vi "Query FTT Data.vi"(8 "error in (no error)":errorcluster, 11 "Main":T1={"Tite"="", "Base path"=path "", "Table"=[], "Stations"=[], "Shield Array"=[], "UPHs"=[], "VISA"={"VISA"="", "baud rate"=9600, "data bits"=8, "parity"=enum."None", "stop bits"=10, "flow control"=0}, "Path"={"roof"=path "", "Config"=path "", "Png"=path ""}, "Ctr"={"DB Dispaly"=refnum, "Error Table"=refnum, "Display"=refnum, "Login"=refnum, "Exit"=refnum, "FTT_Submit"=refnum}, "Login"={"User"="", "Grade"=""}, "information"={"cause"="", "Type"=enum."Inform", "code"=0, "Suroce"="", "Status"=FALSE}, "Local DB"={"Connstr"="", "Database"={"Constr"={"Driver"="", "Server"="", "User"="", "Pwd"="", "Database"=""}, "conn ref"=refnum, "State"=FALSE}}, "Remote DB"={"Connstr"="", "Database"={"Constr"={"Driver"="", "Server"="", "User"="", "Pwd"="", "Database"=""}, "conn ref"=refnum, "State"=FALSE}}, "FTT TV"="", "ExchangeTime"=0, "NVH"="", "EOL Path"=path ""} {"VISA"."flow control" items=["None", "XON/XOFF", "RTS/CTS", "XON/XOFF & RTS/CTS", "DTR/DSR", "XON/XOFF & DTR/DSR"]; "VISA"."stop bits" items=["1.0"=10, "1.5"=15, "2.0"=20]}) -> (0 "error out":errorcluster)   [LabVIEW 2014]
uses:
  Type'def/DB Query.ctl
  <vilib>/Utility/file.llb/Write Delimited Spreadsheet (string).vi
  Type'def/UPH Config.ctl
  VISA/Ctr/VISA Ctr.ctl
  Type'def/Main Ctr Ref.ctl
  Type'def/User Login.ctl
  Database/Ctr/Constr.ctl
  <vilib>/addons/database/Connection.llb/Conn ObjectReference.ctl
  <vilib>/addons/database/NI_Database_API.lvlib
  Database/Ctr/Conneect State.ctl
  Type'def/MainCtr.ctl
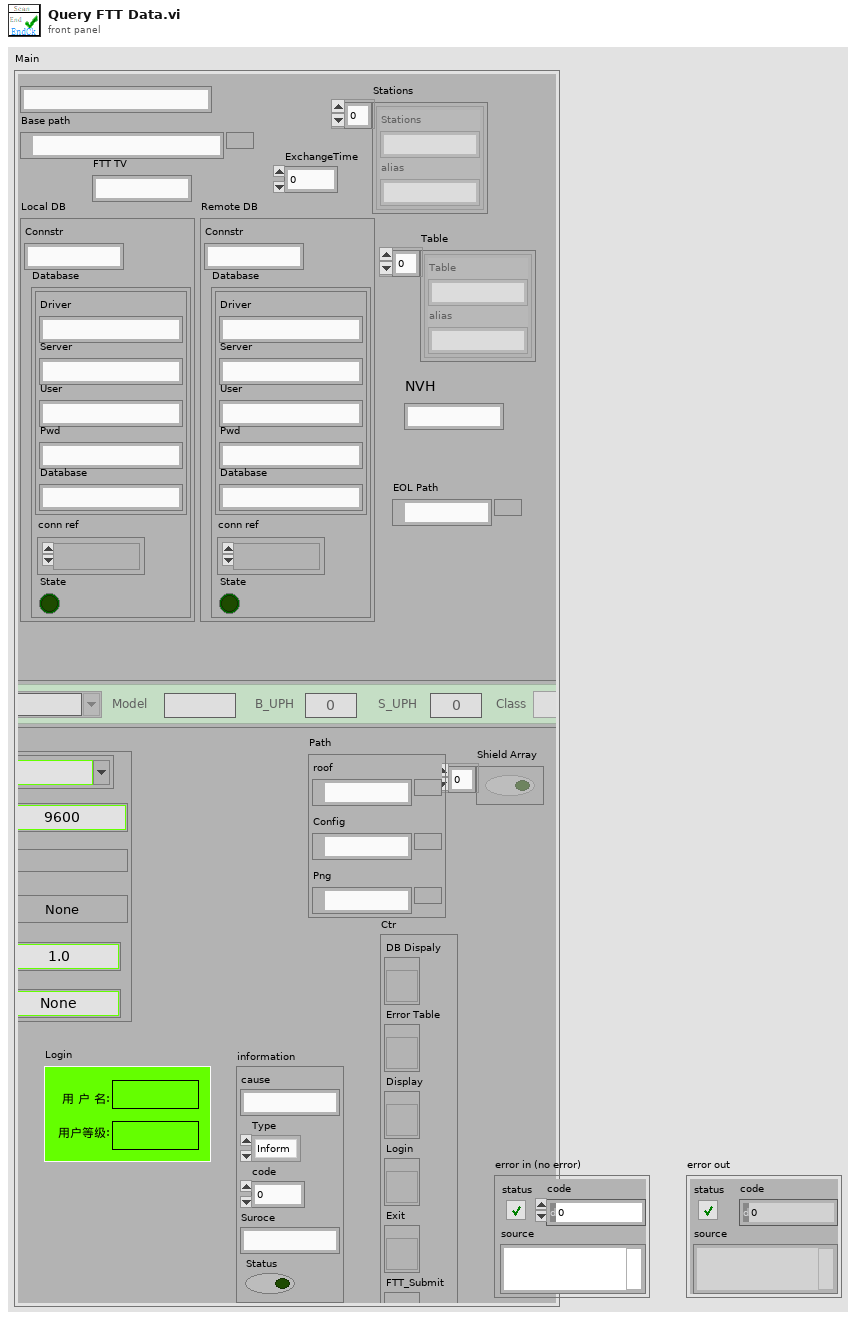
[diagram p1: front panel]
types:
  T1 = typedef "MainCtr.ctl" = cluster{"Tite":string, "Base path":path, "Table":cluster{"Table":string, "alias":string}[], "Stations":cluster{"Stations":string, "alias":string}[], "Shield Array":bool[], "UPHs":T2[], "VISA":T3, "Path":cluster{"roof":path, "Config":path, "Png":path}, "Ctr":T4, "Login":T5, "information":cluster{"cause":string, "Type":enum16{"Inform", "Warning", "Alarm"}, "code":i32, "Suroce":string, "Status":bool}, "Local DB":cluster{"Connstr":string, "Database":T6}, "Remote DB":cluster{"Connstr":string, "Database":T6}, "FTT TV":string, "ExchangeTime":i32, "NVH":string, "EOL Path":path}
  T2 = typedef "UPH Config.ctl" = cluster{"Line_No":string, "Model":string, "B_UPH ":i16, "S_UPH  ":i16, "Class":enum16{"Big", "Small"}}
  T3 = typedef "VISA Ctr.ctl" = cluster{"VISA":refnum<visa-resource-name>, "baud rate":u32, "data bits":u16, "parity":enum16{"None", "Odd", "Even", "Mark", "Space"}, "stop bits":u16, "flow control":u16}
  T4 = typedef "Main Ctr Ref.ctl" = cluster{"DB Dispaly":refnum<vi>, "Error Table":refnum<vi>, "Display":refnum<vi>, "Login":refnum<vi>, "Exit":refnum<vi>, "FTT_Submit":refnum<vi>}
  T5 = typedef "User Login.ctl" = cluster{"User":string, "Grade":string}
  T6 = typedef "Conneect State.ctl" = cluster{"Constr":T7, "conn ref":T8, "State":bool}
  T7 = typedef "Constr.ctl" = cluster{"Driver":string, "Server":string, "User":string, "Pwd":string, "Database":string}
  T8 = typedef "NI_Database_API.lvlib/Conn ObjectReference.ctl" = refnum<k1>
  T9 = cluster{"cause":string, "Type":enum16{"Inform", "Warning", "Alarm"}, "code":i32, "Suroce":string, "Status":bool}
  T10 = typedef "DB Query.ctl" = cluster{"Export":bool, "Query":bool, "Station.No":string, "EndTime":timestamp, "StartTime":timestamp, "FTT":cluster{"FTT":string, "OutLine":string, "FTT Rata":string}, "TableName":string, "List":string[][], "Station":bool, "QTime":enum32{"Online", "Outline"}}
  T11 = cluster{"Main ":T1, "DB Dispaly":T10, "information":cluster{"cause":string, "Type":enum16{"Inform", "Warning", "Alarm"}, "code":i32, "Suroce":string, "Status":bool}, "CmdStr":string, "OnlineStr":string}
  T12 = cluster{"FTT":string, "OutLine":string, "FTT Rata":string}
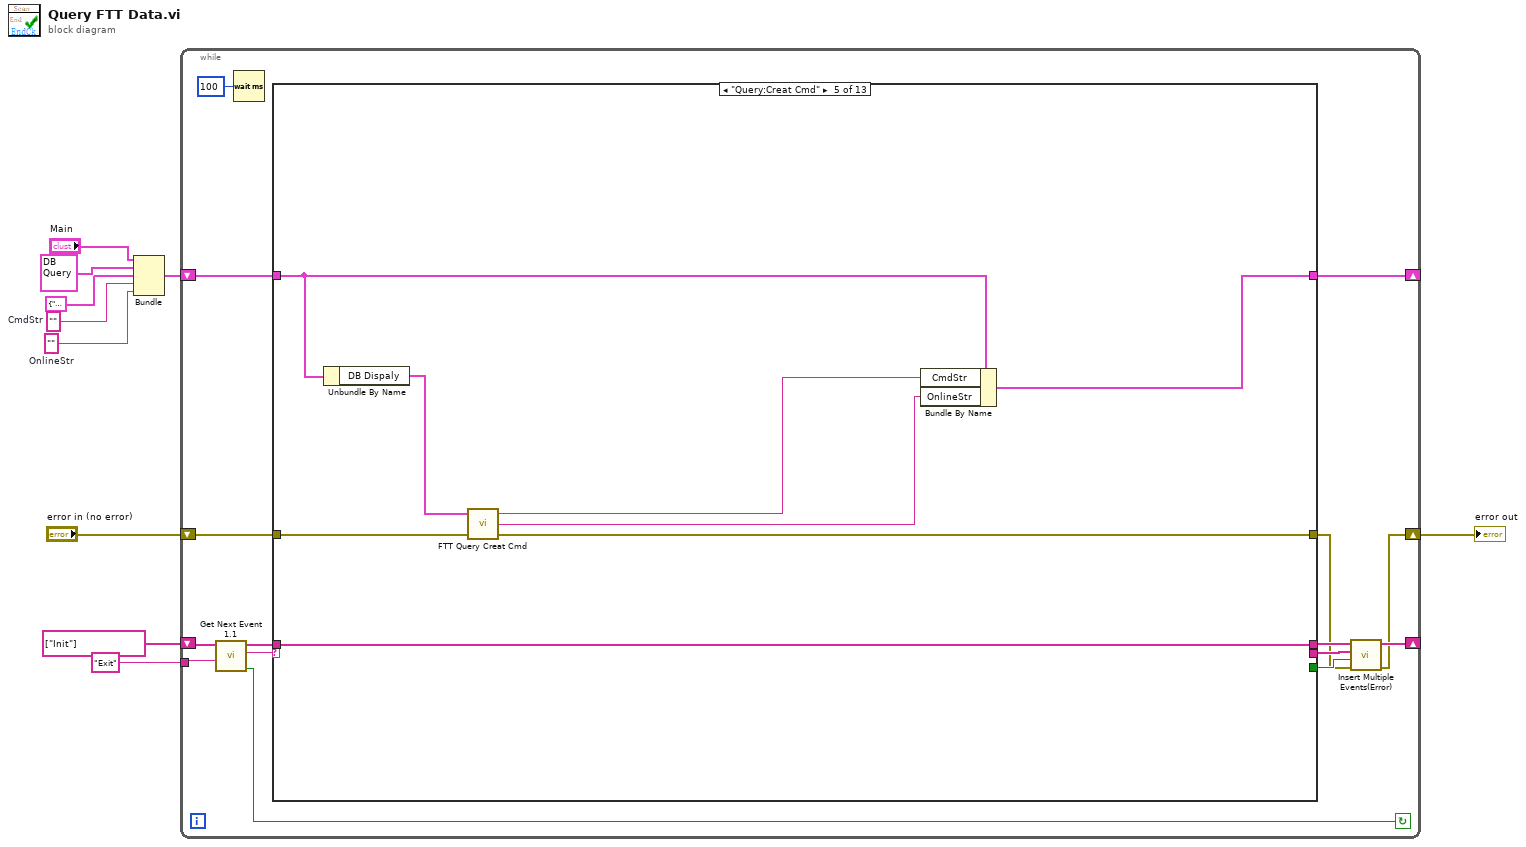
[diagram p0: block diagram]
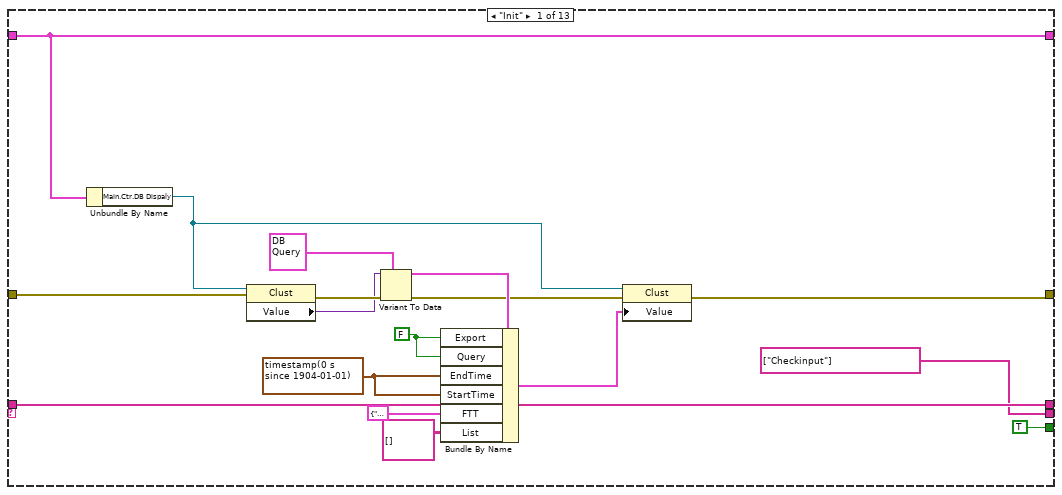
[diagram p2: hidden frame]
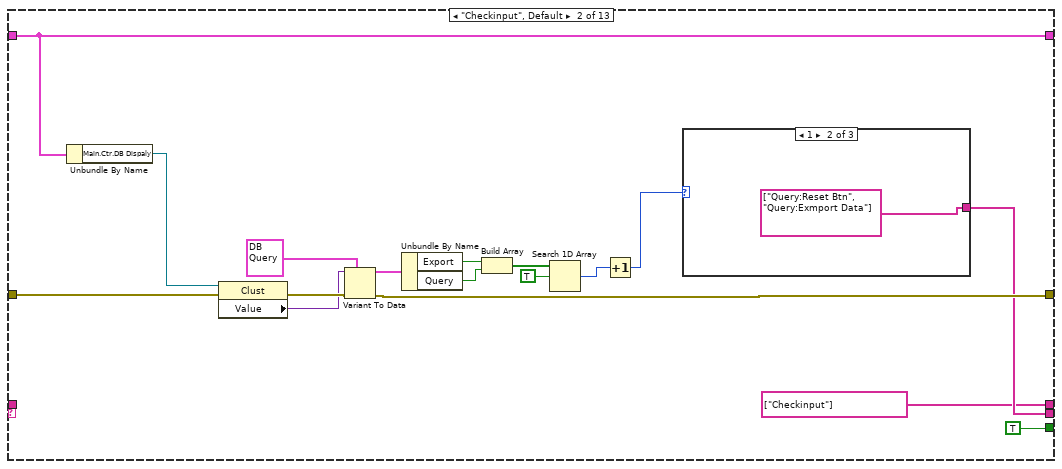
[diagram p3: hidden frame]
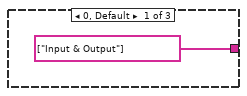
[diagram p4: hidden frame]
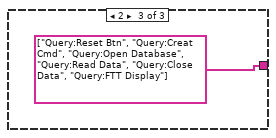
[diagram p5: hidden frame]
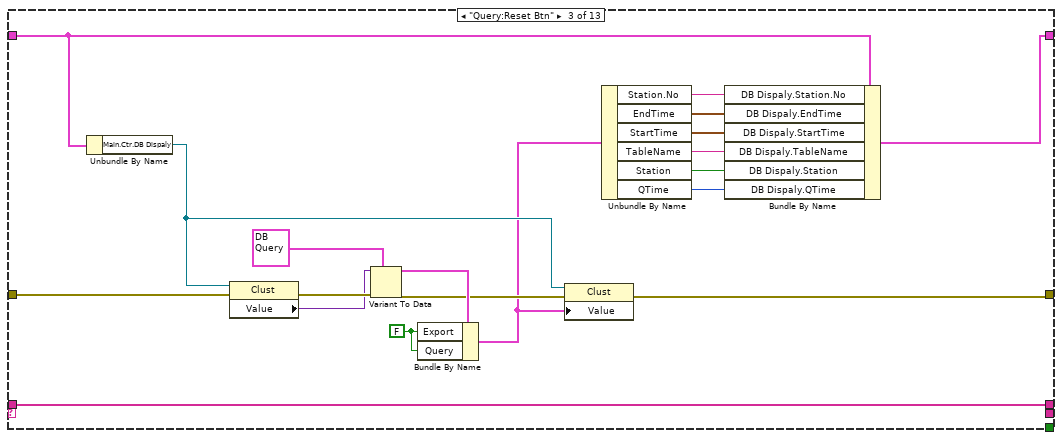
[diagram p6: hidden frame]
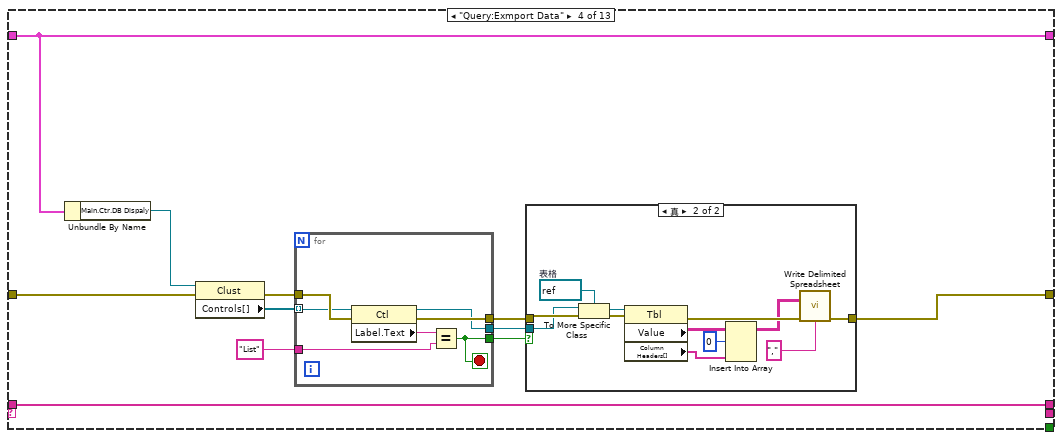
[diagram p7: hidden frame]
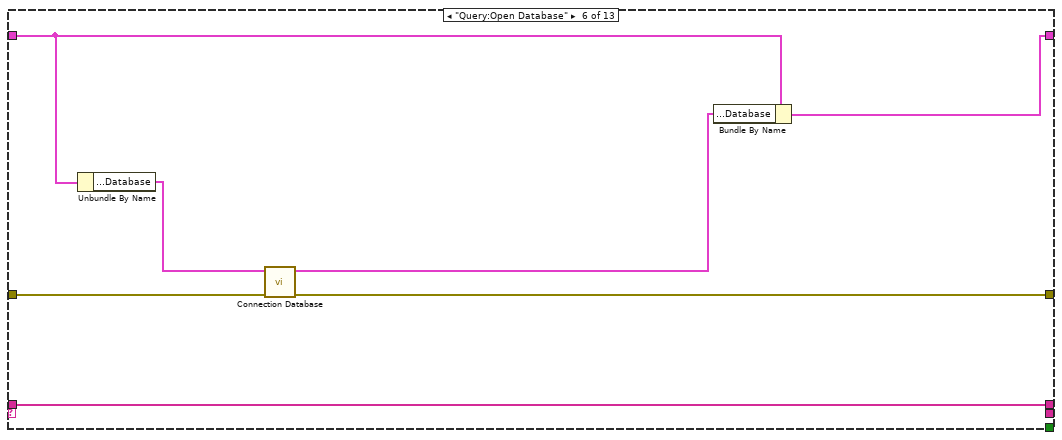
[diagram p9: hidden frame]
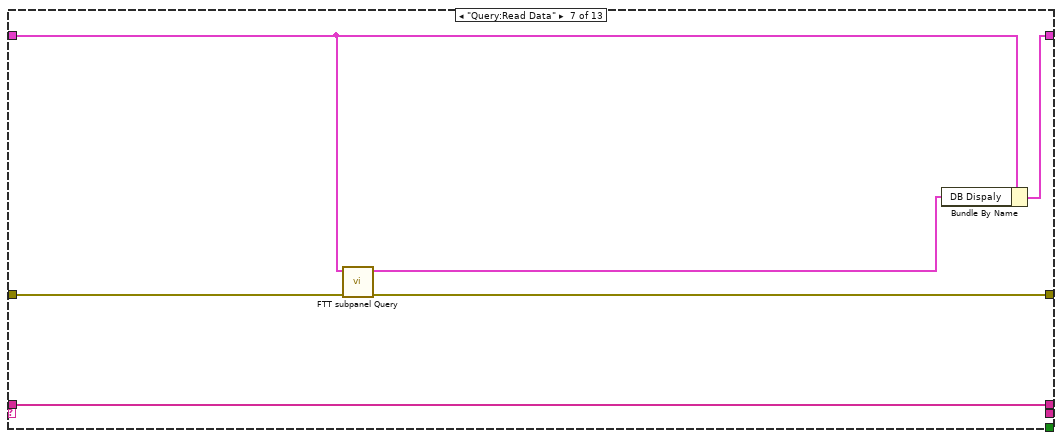
[diagram p10: hidden frame]
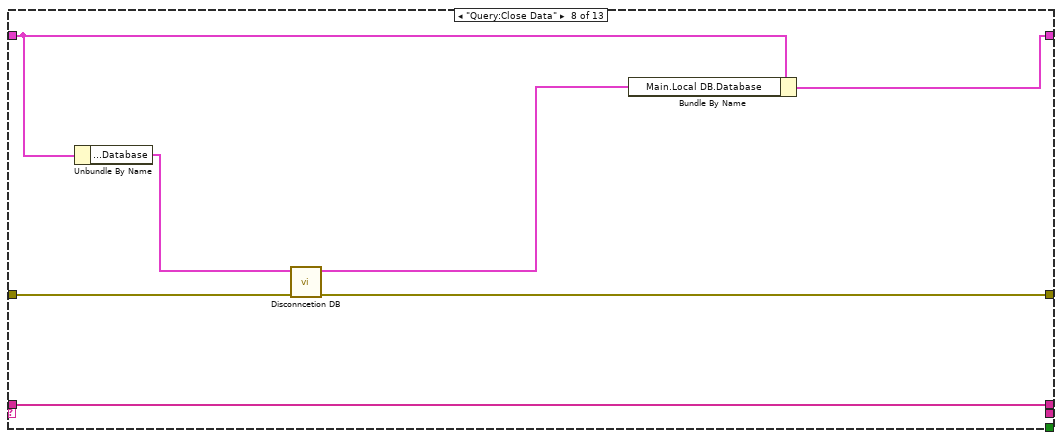
[diagram p11: hidden frame]
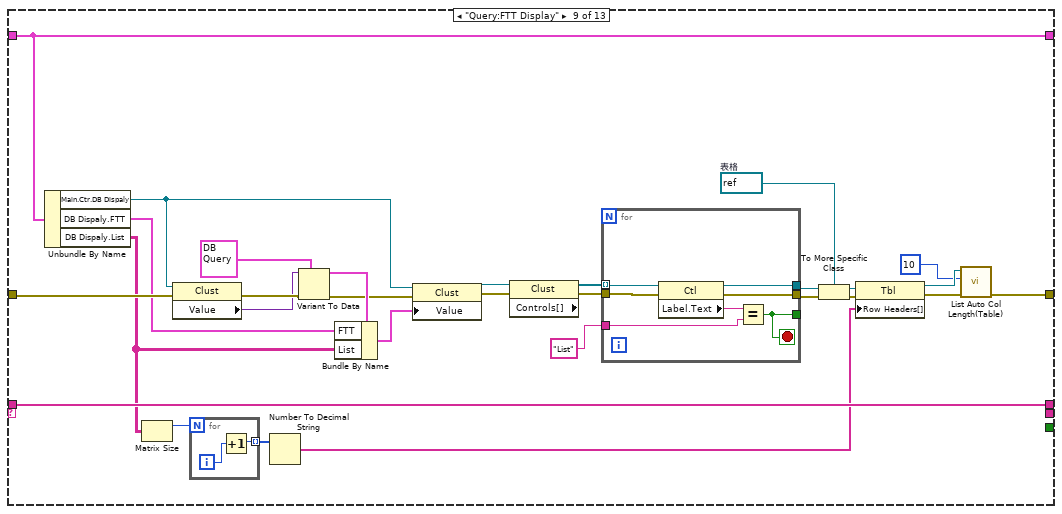
[diagram p12: hidden frame]
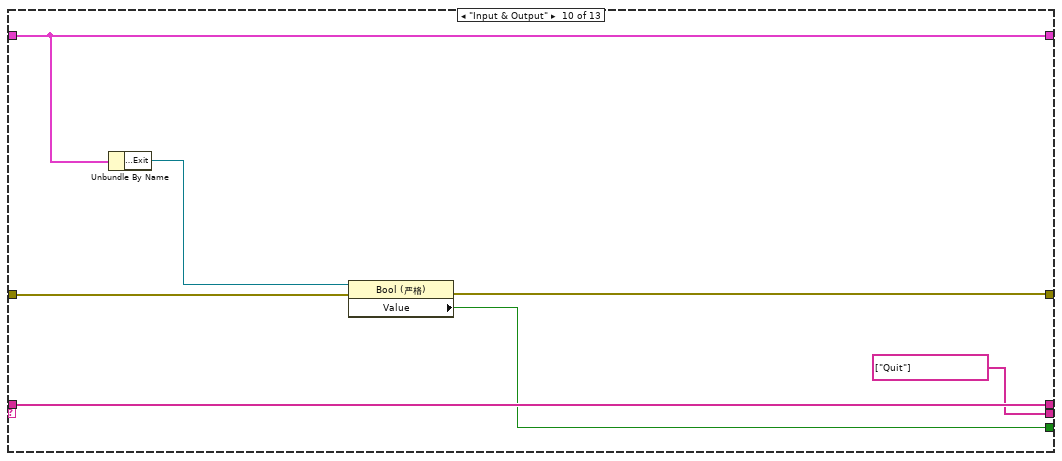
[diagram p13: hidden frame]
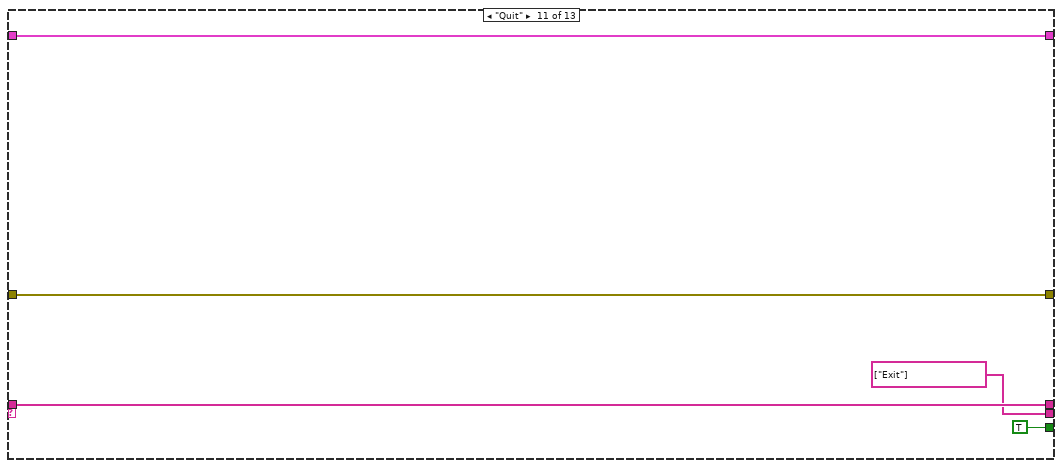
[diagram p14: hidden frame]
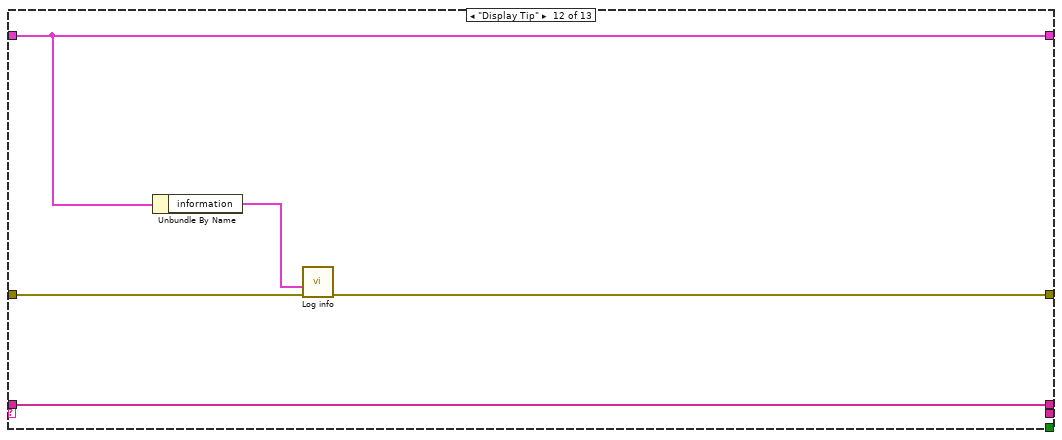
[diagram p15: hidden frame]
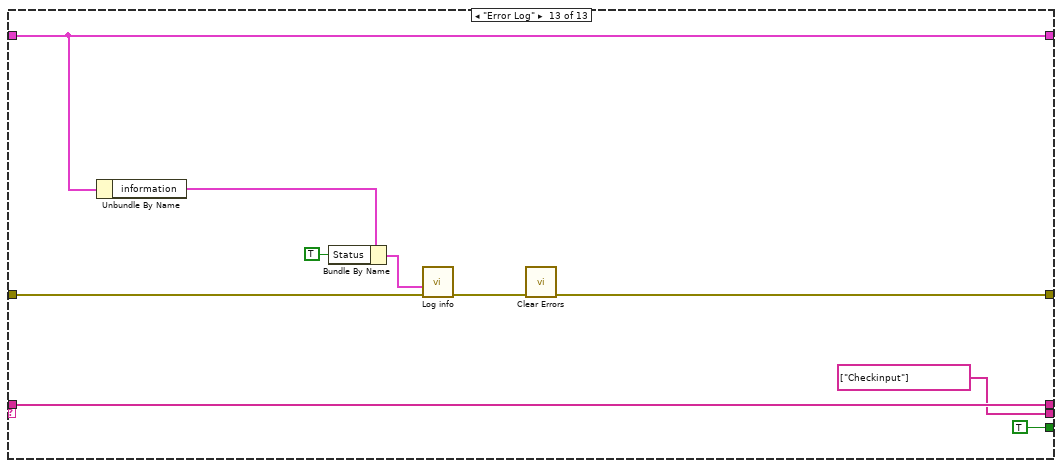
[diagram p16: hidden frame]
diagram:
  w1 = ""  # OnlineStr
  w2 = ""  # CmdStr
  n1 = Bundle("Main"="Main", "DB Dispaly"=T10 {"Export"=FALSE, "Query"=FALSE, "Station.No"="", "EndTime"=timestamp(0 s since 1904-01-01), "StartTime"=timestamp(0 s since 1904-01-01), "FTT"={"FTT"="", "OutLine"="", "FTT Rata"=""}, "TableName"="", "List"=[], "Station"=FALSE, "QTime"=enum."Online"}, "information"=T9 {"cause"="", "Type"=enum."Inform", "code"=0, "Suroce"="", "Status"=FALSE}, "CmdStr"=w2, "OnlineStr"=w1) -> (w7:T11)  [unwired: 1 in]
  n2 = while {
    tunnel: "Exit" ("Exit Event") -> [w22]
    shift-right: [w18] -> _
    shift-left: string[] ["Init"] -> [w23]
    shift-right: [w12] -> w4
    shift-left: "error in (no error)" -> [w21]
    shift-right: [w14] -> _
    shift-left: w7 -> [w19]
    stop <- w24 continue-if-true
    n3 = call "Get Next Event 1.1.vi"("Exit Event"=w22, "event queue in"=w23) -> ("Condition (Exit:F)"=w24:bool, "next event"=w25:string, "event queue out"=w20:string[])  [unwired: 6 in, 1 out]
    n4 = Wait (ms)(milliseconds to wait=u32 100) -> ()  [unwired: 1 out]
    n5 = case shown="\"Query:Creat Cmd\"" w25 {
      tunnel: w21 -> [w40 w57 w81 w91 w118 w127 w131 w139 w165 w184 w189 w195 w205]
      tunnel: w20 -> [w42 _ w72 w86 w119 w121 w133 w140 w169 w181 w188 w191 w198]
      tunnel: w19 -> [w41 w58 w71 w92 w115 w124 w128 w136 w168 w185 w190 w193 w202]
      tunnel: [w28 w51 w73 w82 w117 w126 w130 w138 w153 w182 w189 w194 w203] -> w13
      tunnel: [w42 string[] ["Checkinput"] w72 w86 w119 w121 w133 w140 w169 w181 w188 w191 w198] -> w17
      tunnel: [TRUE ("Insert all? (T)") TRUE ("Insert all? (T)") _ _ _ _ _ _ _ w180 TRUE ("Insert all? (T)") _ TRUE ("Insert all? (T)")] -> w16
      tunnel: [string[] ["Checkinput"] w44 _ _ _ _ _ _ _ string[] ["Quit"] string[] ["Exit"] _ string[] ["Checkinput"]] -> w15
      tunnel: [w41 w58 w70 w92 w114 w122 w132 w134 w168 w185 w190 w193 w202] -> w14
      frame "Init" {
        w34 = timestamp(0 s since 1904-01-01)
        w35 = FALSE
        n6 = Unbundle By Name(w41) -> ("Main.Ctr.DB Dispaly"=w30:refnum<vi>)
        n7 = property class="Clust"(reference=w30, error in=w40) -> (error out=w39:errorcluster, "Value"=w38:variant)  [unwired: 1 out]
        n8 = Variant To Data(error in=w39, type=T10 {"Export"=FALSE, "Query"=FALSE, "Station.No"="", "EndTime"=timestamp(0 s since 1904-01-01), "StartTime"=timestamp(0 s since 1904-01-01), "FTT"={"FTT"="", "OutLine"="", "FTT Rata"=""}, "TableName"="", "List"=[], "Station"=FALSE, "QTime"=enum."Online"} ("DB Dispaly"), Variant=w38) -> (data=w36:T10, error out=w31:errorcluster)
        n9 = Bundle By Name(cluster=w36, "Export"=w35, "Query"=w35, "EndTime"=w34, "StartTime"=w34, "FTT"=T12 {"FTT"="", "OutLine"="", "FTT Rata"=""}, "List"=string[][] []) -> (w29:T10)
        n10 = property class="Clust"(reference=w30, error in=w31, "Value"=w29) -> (error out=w28:errorcluster)  [unwired: 1 out]
      }
      frame "Checkinput", Default {
        n11 = Unbundle By Name(w58) -> ("Main.Ctr.DB Dispaly"=w56:refnum<vi>)
        n12 = property class="Clust"(reference=w56, error in=w57) -> (error out=w55:errorcluster, "Value"=w54:variant)  [unwired: 1 out]
        n13 = Variant To Data(error in=w55, type=T10 {"Export"=FALSE, "Query"=FALSE, "Station.No"="", "EndTime"=timestamp(0 s since 1904-01-01), "StartTime"=timestamp(0 s since 1904-01-01), "FTT"={"FTT"="", "OutLine"="", "FTT Rata"=""}, "TableName"="", "List"=[], "Station"=FALSE, "QTime"=enum."Online"} ("DB Dispaly"), Variant=w54) -> (data=w52:T10, error out=w51:errorcluster)
        n14 = Unbundle By Name(w52) -> ("Export"=w50:bool, "Query"=w49:bool)
        n15 = Build Array(w50, w49) -> (w48:bool[])
        n16 = Search 1D Array(1D array=w48, element=TRUE) -> (index of element=w46:i32)  [unwired: 1 in]
        n17 = Increment(x=w46) -> (x+1=w45:i32)
        n18 = case shown="1" w45 {
          tunnel: [string[] ["Input & Output"] string[] ["Query:Reset Btn", "Query:Exmport Data"] string[] ["Query:Reset Btn", "Query:Creat Cmd", "Query:Open Database", "Query:Read Data", "Query:Close Data", "Query:FTT Display"]] -> w44
          frame 0, Default {
          }
          frame 1 {
          }
          frame 2 {
          }
        }
      }
      frame "Query:Reset Btn" {
        w76 = FALSE
        n19 = Unbundle By Name(w71) -> ("Main.Ctr.DB Dispaly"=w74:refnum<vi>)
        n20 = property class="Clust"(reference=w74, error in=w81) -> (error out=w80:errorcluster, "Value"=w79:variant)  [unwired: 1 out]
        n21 = Variant To Data(error in=w80, type=T10 {"Export"=FALSE, "Query"=FALSE, "Station.No"="", "EndTime"=timestamp(0 s since 1904-01-01), "StartTime"=timestamp(0 s since 1904-01-01), "FTT"={"FTT"="", "OutLine"="", "FTT Rata"=""}, "TableName"="", "List"=[], "Station"=FALSE, "QTime"=enum."Online"} ("DB Dispaly"), Variant=w79) -> (data=w77:T10, error out=w75:errorcluster)
        n22 = Bundle By Name(cluster=w77, "Export"=w76, "Query"=w76) -> (w69:T10)
        n23 = property class="Clust"(reference=w74, error in=w75, "Value"=w69) -> (error out=w73:errorcluster)  [unwired: 1 out]
        n24 = Unbundle By Name(w69) -> ("Station.No"=w68:string, "EndTime"=w67:timestamp, "StartTime"=w66:timestamp, "TableName"=w65:string, "Station"=w64:bool, "QTime"=w63:enum32{"Online", "Outline"})
        n25 = Bundle By Name(cluster=w71, "DB Dispaly.Station.No"=w68, "DB Dispaly.EndTime"=w67, "DB Dispaly.StartTime"=w66, "DB Dispaly.TableName"=w65, "DB Dispaly.Station"=w64, "DB Dispaly.QTime"=w63) -> (w70:T11)
      }
      frame "Query:Exmport Data" {
        n26 = Unbundle By Name(w92) -> ("Main.Ctr.DB Dispaly"=w90:refnum<vi>)
        n27 = property class="Clust"(reference=w90, error in=w91) -> (error out=w87:errorcluster, "Controls[]"=w89:refnum<vi>[])  [unwired: 1 out]
        n28 = for {
          tunnel: w89 -> [w108] mode=indexing
          tunnel: "List" -> [w111]
          tunnel: w87 -> [w112]
          tunnel: [w106] -> w84
          tunnel: [w109] -> w85
          tunnel: [w107] -> w83
          stop <- w109 stop-if-true
          n29 = property class="Ctl"(reference=w108, error in=w112) -> (reference out=w106:refnum<vi>, error out=w107:errorcluster, "Label.Text"=w110:string)
          n30 = Equal?(x=w110, y=w111) -> (x = y?=w109:bool)
        }
        n31 = case shown="真" w85 {
          tunnel: w84 -> [_ w104]
          tunnel: w83 -> [w93 w105]
          tunnel: [w93 w94] -> w82
          frame False {
          }
          frame True {
            w101 = refnum<vi> refnum  # 表格
            n32 = To More Specific Class(target class=w101, reference=w104, error in=w105) -> (specific class reference=w102:refnum<vi>, error out=w103:errorcluster)
            n33 = property class="Tbl"(reference=w102, error in=w103) -> (error out=w97:errorcluster, "Value"=w100:string[][], "Column Headers[]"=w98:string[])  [unwired: 1 out]
            n34 = Insert Into Array(array=w100, index (row)=0, new element=w98) -> (w96:string[][])  [unwired: 1 in]
            n35 = call-poly <vilib>:"Write Delimited Spreadsheet.vi"("2D data"=w96, "error in (no error)"=w97, "delimiter (\\t)"="," ("delimiter (\\t)")) -> ("error out"=w94:errorcluster)  [unwired: 11 in, 1 out]
          }
        }
      }
      frame "Query:Creat Cmd" {
        n36 = Unbundle By Name(w115) -> ("DB Dispaly"=w120:T10)
        n37 = call "FTT Query Creat Cmd.vi"("error in (no error)"=w118, "DB Dispaly"=w120) -> ("error out"=w117:errorcluster, "Strs"=w113:string, "Str"=w116:string)  [unwired: 1 in]
        n38 = Bundle By Name(cluster=w115, "CmdStr"=w116, "OnlineStr"=w113) -> (w114:T11)
      }
      frame "Query:Open Database" {
        n39 = Unbundle By Name(w124) -> ("Main.Local DB.Database"=w125:T6)
        n40 = call "Connection Database.vi"("error in (no error)"=w127, "Connncet State"=w125) -> ("error out"=w126:errorcluster, "Connncet State out"=w123:T6)  [unwired: 8 in]
        n41 = Bundle By Name(cluster=w124, "Main.Local DB.Database"=w123) -> (w122:T11)
      }
      frame "Query:Read Data" {
        n42 = call "FTT subpanel Query.vi"("error in (no error)"=w131, "Cluster"=w128) -> ("error out"=w130:errorcluster, "DB Dispaly"=w129:T10)  [unwired: 8 in]
        n43 = Bundle By Name(cluster=w128, "DB Dispaly"=w129) -> (w132:T11)
      }
      frame "Query:Close Data" {
        n44 = Unbundle By Name(w136) -> ("Main.Local DB.Database"=w137:T6)
        n45 = call "Disconncetion DB.vi"("error in (no error)"=w139, "Connncet State"=w137) -> ("error out"=w138:errorcluster, "Connect State"=w135:T6)  [unwired: 8 in]
        n46 = Bundle By Name(cluster=w136, "Main.Local DB.Database"=w135) -> (w134:T11)
      }
      frame "Query:FTT Display" {
        w146 = refnum<vi> refnum  # 表格
        n47 = Unbundle By Name(w168) -> ("Main.Ctr.DB Dispaly"=w160:refnum<vi>, "DB Dispaly.FTT"=w162:T12, "DB Dispaly.List"=w141:string[][])
        n48 = Matrix Size(0:w141) -> (1:w152:i32)  [unwired: 1 out]
        n49 = property class="Clust"(reference=w160, error in=w165) -> (error out=w167:errorcluster, "Value"=w166:variant)  [unwired: 1 out]
        n50 = for {
          N: w152 -> [_]
          tunnel: [w170] -> w151 mode=indexing
          i -> [w171]
          n51 = Increment(x=w171) -> (x+1=w170:i32)
        }
        n52 = Number To Decimal String(number=w151) -> (decimal integer string=w145:string[])  [unwired: 1 in]
        n53 = Variant To Data(error in=w167, type=T10 {"Export"=FALSE, "Query"=FALSE, "Station.No"="", "EndTime"=timestamp(0 s since 1904-01-01), "StartTime"=timestamp(0 s since 1904-01-01), "FTT"={"FTT"="", "OutLine"="", "FTT Rata"=""}, "TableName"="", "List"=[], "Station"=FALSE, "QTime"=enum."Online"} ("DB Dispaly"), Variant=w166) -> (data=w163:T10, error out=w161:errorcluster)
        n54 = Bundle By Name(cluster=w163, "FTT"=w162, "List"=w141) -> (w159:T10)
        n55 = property class="Clust"(reference=w160, error in=w161, "Value"=w159) -> (reference out=w154:refnum<vi>, error out=w155:errorcluster)
        n56 = property class="Clust"(reference=w154, error in=w155) -> (error out=w156:errorcluster, "Controls[]"=w158:refnum<vi>[])  [unwired: 1 out]
        n57 = for {
          tunnel: w158 -> [w174] mode=indexing
          tunnel: "List" -> [w177]
          tunnel: w156 -> [w178]
          tunnel: [w172] -> w148
          tunnel: [w175] -> _
          tunnel: [w173] -> w149
          stop <- w175 stop-if-true
          n58 = property class="Ctl"(reference=w174, error in=w178) -> (reference out=w172:refnum<vi>, error out=w173:errorcluster, "Label.Text"=w176:string)
          n59 = Equal?(x=w176, y=w177) -> (x = y?=w175:bool)
        }
        n60 = To More Specific Class(target class=w146, reference=w148, error in=w149) -> (specific class reference=w147:refnum<vi>, error out=w150:errorcluster)
        n61 = property class="Tbl"(reference=w147, error in=w150, "Row Headers[]"=w145) -> (reference out=w143:refnum<vi>, error out=w144:errorcluster)
        n62 = call "List Auto Col Length(Table).vi"("错误输入（无错误）"=w144, "Rows"=10, "Comm ref"=w143) -> ("错误输出"=w153:errorcluster)  [unwired: 7 in, 1 out]
      }
      frame "Input & Output" {
        n63 = Unbundle By Name(w185) -> ("Main.Ctr.Exit"=w183:refnum<vi>)
        n64 = property class="Bool (严格)"(reference=w183, error in=w184) -> (error out=w182:errorcluster, "Value"=w180:bool)  [unwired: 1 out]
      }
      frame "Quit" {
      }
      frame "Display Tip" {
        n65 = Unbundle By Name(w193) -> ("information"=w192:T9)
        n66 = call "Log info.vi"("error in (no error)"=w195, "information"=w192) -> ("error out"=w194:errorcluster)  [unwired: 8 in, 1 out]
      }
      frame "Error Log" {
        n67 = Unbundle By Name(w202) -> ("information"=w201:T9)
        n68 = Bundle By Name(cluster=w201, "Status"=TRUE) -> (w200:T9)
        n69 = call "Log info.vi"("error in (no error)"=w205, "information"=w200) -> ("error out"=w204:errorcluster)  [unwired: 8 in, 1 out]
        n70 = call <vilib>:"Clear Errors.vi"("error in (no error)"=w204) -> ("error out"=w203:errorcluster)  [unwired: 5 in, 1 out]
      }
    }
    n71 = call "Insert Multiple Events(Error).vi"("error in (no error)"=w13, "Insert all? (T)"=w16, "Events to Insert"=w15, "Event queue in"=w17) -> ("error out"=w12:errorcluster, "Event queue out"=w18:string[])  [unwired: 6 in]
  }
  "error out" <- w4
